vi "Mirror_GUI.vi"(10 "stop 2":refnum<vi>, 11 "GUI_cluster":T1={"Sub Panel"=refnum, "GUIdevice"="Bella_LP_Mode", "CtlRef"=refnum, "user event out"=refnum}) -> ()   [LabVIEW 2011]
uses:
  Controls/GUI_cluster.ctl
  Controls/eventtypdef.ctl
  GUI_Template/GUI_master/tcp new data cluster.ctl
  General-Controler/firstCall_TypDef.ctl
panel:
  out "UDP error message":string
  out "status ref":refnum<vi>[](array[refnum])
  out "pathRef":refnum<vi>[](array[refnum])
  in  "pushSave":bool
  out "Page Label":string="StagingTRA1"
  in  "save::4":bool caption="save"
  in  "save::3":bool caption="save"
  in  "save::2":bool caption="save"
  in  "save::1":bool caption="save"
  in  "LocalSavingPath::4":path=path "Z:/5_resources/StagingResources/TRAposition/testNEW" caption="LocalSavingPath::1"
  in  "LocalSavingPath::3":path=path "Z:/5_resources/StagingResources/TRAposition/testNEW" caption="LocalSavingPath::1"
  in  "LocalSavingPath::2":path=path "Z:/5_resources/StagingResources/TRAposition/testNEW" caption="LocalSavingPath::1"
  in  "LocalSavingPath::1":path=path "Z:/5_resources/StagingResources/TRAposition/testNEW"
  in  "save":bool
  out "GUIdevice 3":string="StagingTRA3"
  out "GUIdevice 4":string="TREX TRA1"
  out "error out":errorcluster
  out "GUIdevice 2":string="StagingTRA2"
  in  "Tab Control":T2(tab)
  in  "StepSize::1":dbl=0.01 caption="StepSize" min=-1.0 max=1.0 format="%#_2p"
  in  "Cluster 20":T3
  in  "Y":T4={"position::1"=2.74161, "Channel::1"=enum."Axis 2", "Status::1"=enum."DISABLE"} {"position::1" min=0.0 max=6.0 format="%#_8g"}
  in  "X":T5={"position::1"=3.02685, "Channel::1"=enum."Axis 1", "Status::1"=enum."DISABLE"} {"position::1" min=0.0 max=6.0 format="%#_8g"}
  in  "Cluster 40":T6
  in  "Cluster 50":T7
  in  "Cluster 30":T8
  out "device status::1":string="Initialized" caption="Device status"
  in  "<command>::1":bool
  in  "StepSize::2":dbl=0.01 caption="StepSize" min=-1.0 max=1.0 format="%#_2p"
  in  "Cluster 23":T9
  in  "Y":T10={"position::2"=3.24237, "Channel::2"=enum."Axis 2", "Status::2"=enum."DISABLE"} {"position::2" min=0.0 max=6.0 format="%#_8g"}
  in  "X":T11={"position::2"=2.27011, "Channel::2"=enum."Axis 1", "Status::2"=enum."DISABLE"} {"position::2" min=0.0 max=6.0 format="%#_8g"}
  in  "Cluster 43":T12
  in  "Cluster 53":T13
  in  "Cluster 33":T14
  out "device status::2":string="Initialized" caption="Device status"
  in  "<command>::2":bool
  in  "StepSize::3":dbl=0.01 caption="StepSize" min=-1.0 max=1.0 format="%#_2p"
  in  "Cluster 22":T15
  in  "Y":T16={"position::3"=5.00224, "Channel::3"=enum."Axis 2", "Status::3"=enum."DISABLE"} {"position::3" min=0.0 max=0.0 format="%#_8g"}
  in  "X":T17={"position::3"=1.52721, "Channel::3"=enum."Axis 1", "Status::3"=enum."DISABLE"} {"position::3" min=0.0 max=0.0 format="%#_8g"}
  in  "Cluster 42":T18
  in  "Cluster 52":T19
  in  "Cluster 32":T20
  out "device status::3":string="Initialized" caption="Device status"
  in  "<command>::3":bool
  in  "StepSize::4":dbl=0.01 caption="StepSize" min=-1.0 max=1.0 format="%#_2p"
  in  "Cluster 21":T21
  in  "Y":T22={"position::4"=4.68088, "Channel::4"=enum."Axis 2", "Status::4"=enum."DISABLE"} {"position::4" min=0.0 max=6.0 format="%#_8g"}
  in  "X":T23={"position::4"=0.99394, "Channel::4"=enum."Axis 1", "Status::4"=enum."DISABLE"} {"position::4" min=0.0 max=6.0 format="%#_8g"}
  in  "Cluster 41":T24
  in  "Cluster 51":T25
  in  "Cluster 31":T26
  out "device status::4":string="Initialized" caption="Device status"
  in  "<command>::4":bool
  in  "Mirror":T27(ring)
  out "GUIdevice 1":string="StagingTRA1"
  in  "stop":bool
  in  "Refresh Button":bool
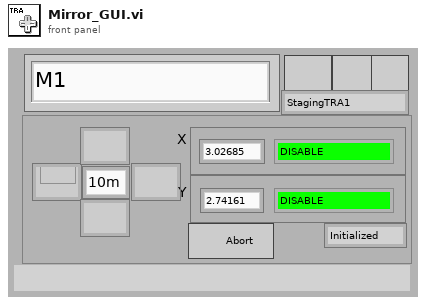
[diagram p1: front panel]
types:
  T1 = typedef "GUI_cluster.ctl" = cluster{"Sub Panel":refnum<vi>, "GUIdevice":string, "CtlRef":refnum<vi>, "user event out":refnum<user-event>}
  T2 = enum32{"StagingTRA1", "StagingTRA2", "StagingTRA3", "TREX TRA1"}
  T3 = cluster{"relativeMovePos::1":bool, "Channel::1":enum16{"Axis 1", "Axis 3", "Axis 5"}}
  T4 = cluster{"position::1":dbl, "Channel::1":enum16{"Axis 2", "Axis 4", "Axis 6"}, "Status::1":enum16{"NOT REFERENCED", "CONFIGURATION", "HOMING", "MOVING", "READY", "DISABLE", "JOGGING"}}
  T5 = cluster{"position::1":dbl, "Channel::1":enum16{"Axis 1", "Axis 3", "Axis 5"}, "Status::1":enum16{"NOT REFERENCED", "CONFIGURATION", "HOMING", "MOVING", "READY", "DISABLE", "JOGGING"}}
  T6 = cluster{"relativeMovePos::1":bool, "Channel::1":enum16{"Axis 2", "Axis 4", "Axis 6"}}
  T7 = cluster{"relativeMoveNeg::1":bool, "Channel::1":enum16{"Axis 2", "Axis 4", "Axis 6"}}
  T8 = cluster{"relativeMoveNeg::1":bool, "Channel::1":enum16{"Axis 1", "Axis 3", "Axis 5"}}
  T9 = cluster{"relativeMovePos::2":bool, "Channel::2":enum16{"Axis 1", "Axis 3", "Axis 5"}}
  T10 = cluster{"position::2":dbl, "Channel::2":enum16{"Axis 2", "Axis 4", "Axis 6"}, "Status::2":enum16{"NOT REFERENCED", "CONFIGURATION", "HOMING", "MOVING", "READY", "DISABLE", "JOGGING"}}
  T11 = cluster{"position::2":dbl, "Channel::2":enum16{"Axis 1", "Axis 3", "Axis 5"}, "Status::2":enum16{"NOT REFERENCED", "CONFIGURATION", "HOMING", "MOVING", "READY", "DISABLE", "JOGGING"}}
  T12 = cluster{"relativeMovePos::2":bool, "Channel::2":enum16{"Axis 2", "Axis 4", "Axis 6"}}
  T13 = cluster{"relativeMoveNeg::2":bool, "Channel::2":enum16{"Axis 2", "Axis 4", "Axis 6"}}
  T14 = cluster{"relativeMoveNeg::2":bool, "Channel::2":enum16{"Axis 1", "Axis 3", "Axis 5"}}
  T15 = cluster{"relativeMovePos::3":bool, "Channel::3":enum16{"Axis 1", "Axis 3", "Axis 5"}}
  T16 = cluster{"position::3":dbl, "Channel::3":enum16{"Axis 2", "Axis 4", "Axis 6"}, "Status::3":enum16{"NOT REFERENCED", "CONFIGURATION", "HOMING", "MOVING", "READY", "DISABLE", "JOGGING"}}
  T17 = cluster{"position::3":dbl, "Channel::3":enum16{"Axis 1", "Axis 3", "Axis 5"}, "Status::3":enum16{"NOT REFERENCED", "CONFIGURATION", "HOMING", "MOVING", "READY", "DISABLE", "JOGGING"}}
  T18 = cluster{"relativeMovePos::3":bool, "Channel::3":enum16{"Axis 2", "Axis 4", "Axis 6"}}
  T19 = cluster{"relativeMoveNeg::3":bool, "Channel::3":enum16{"Axis 2", "Axis 4", "Axis 6"}}
  T20 = cluster{"relativeMoveNeg::3":bool, "Channel::3":enum16{"Axis 1", "Axis 3", "Axis 5"}}
  T21 = cluster{"relativeMovePos::4":bool, "Channel::4":enum16{"Axis 1", "Axis 3", "Axis 5"}}
  T22 = cluster{"position::4":dbl, "Channel::4":enum16{"Axis 2", "Axis 4", "Axis 6"}, "Status::4":enum16{"NOT REFERENCED", "CONFIGURATION", "HOMING", "MOVING", "READY", "DISABLE", "JOGGING"}}
  T23 = cluster{"position::4":dbl, "Channel::4":enum16{"Axis 1", "Axis 3", "Axis 5"}, "Status::4":enum16{"NOT REFERENCED", "CONFIGURATION", "HOMING", "MOVING", "READY", "DISABLE", "JOGGING"}}
  T24 = cluster{"relativeMovePos::4":bool, "Channel::4":enum16{"Axis 2", "Axis 4", "Axis 6"}}
  T25 = cluster{"relativeMoveNeg::4":bool, "Channel::4":enum16{"Axis 2", "Axis 4", "Axis 6"}}
  T26 = cluster{"relativeMoveNeg::4":bool, "Channel::4":enum16{"Axis 1", "Axis 3", "Axis 5"}}
  T27 = enum16{"M1", "BS", "M3", "OAP1", "M4", "OAP2", "M5", "n/a", "n/a ", "M20", "SIM", "M22"}
  T28 = typedef "eventtypdef.ctl" = cluster{"label":string, "Sub Panel":refnum<vi>, "CtlRef":refnum<vi>, "This VI":refnum<vi>}
  T29 = typedef "tcp new data cluster.ctl" = cluster{"EventEnum":enum16{"new data", "connection status update"}, "Device name":string}
  T30 = typedef "firstCall_TypDef.ctl" = enum16{"reset", "read"}
  T31 = typedef "LVFontTypeDef.ctl" = cluster{"Font Name":string, "Size":u16, "Bold":bool, "Italic":bool, "Underline":bool, "Strikeout":bool, "Color":u32}
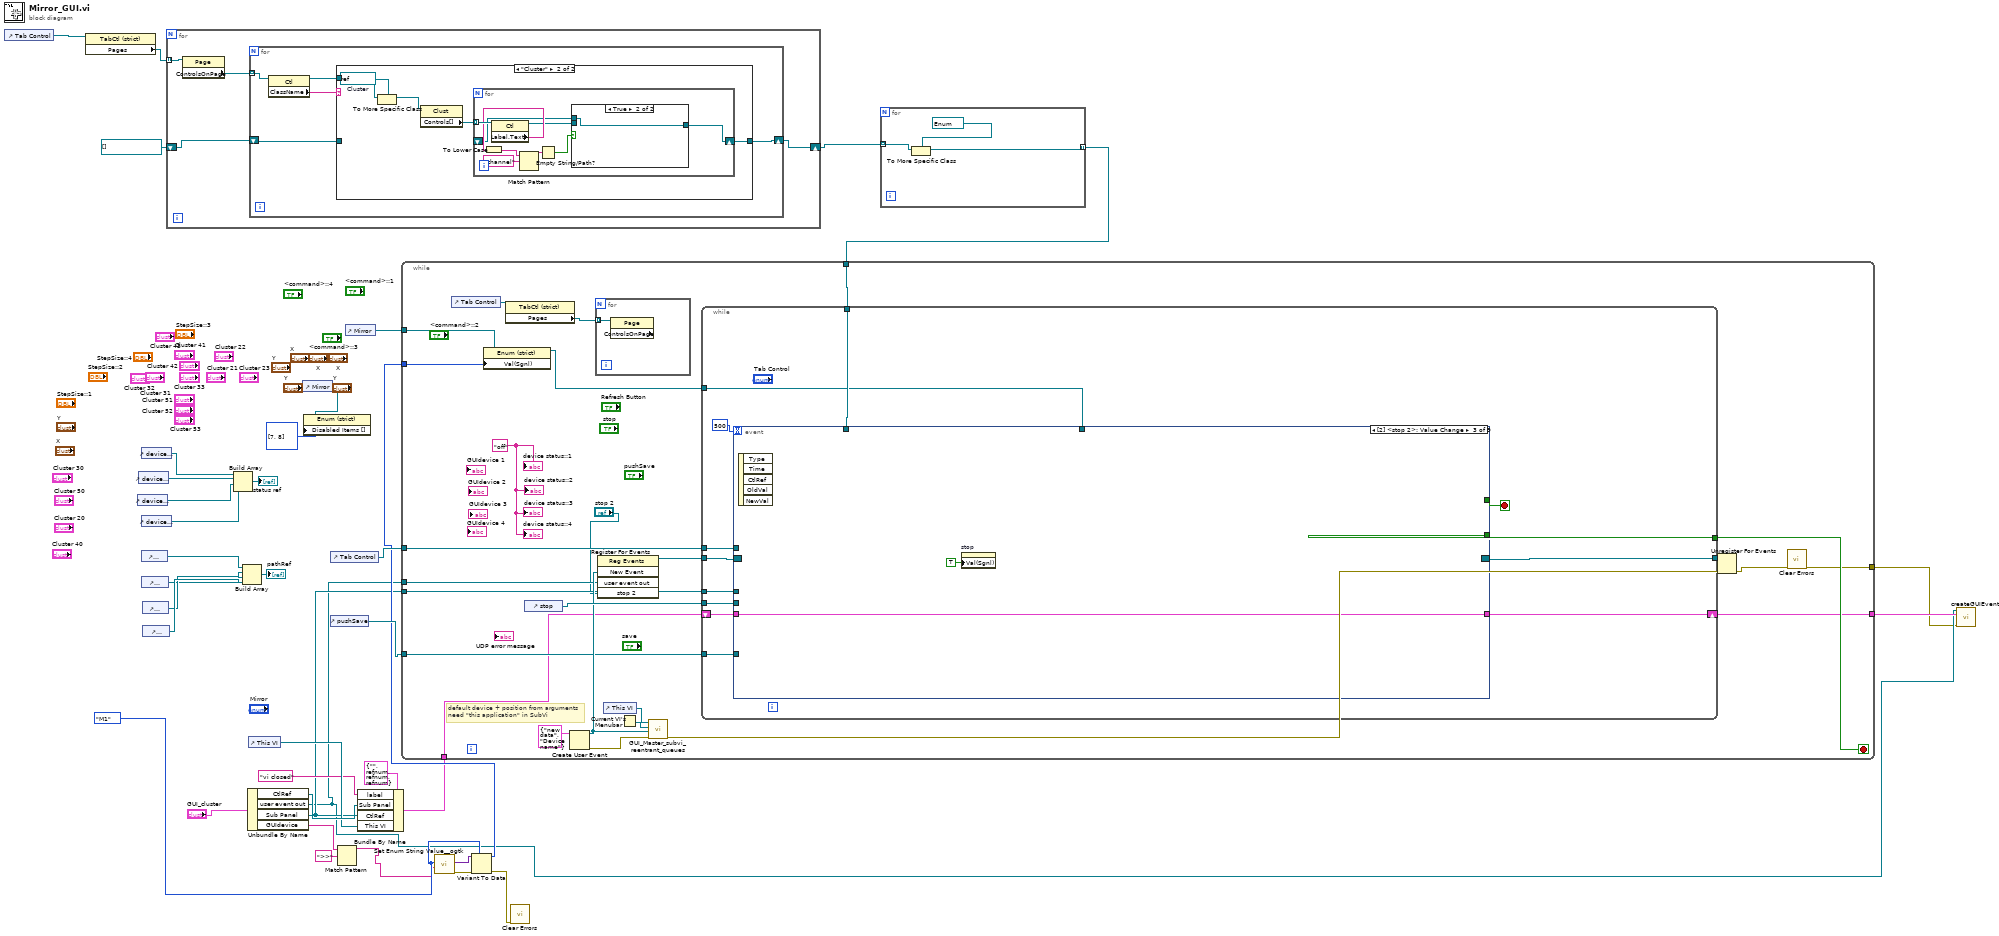
[diagram p0: block diagram]
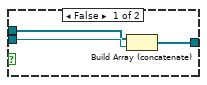
[diagram p3: hidden frame]
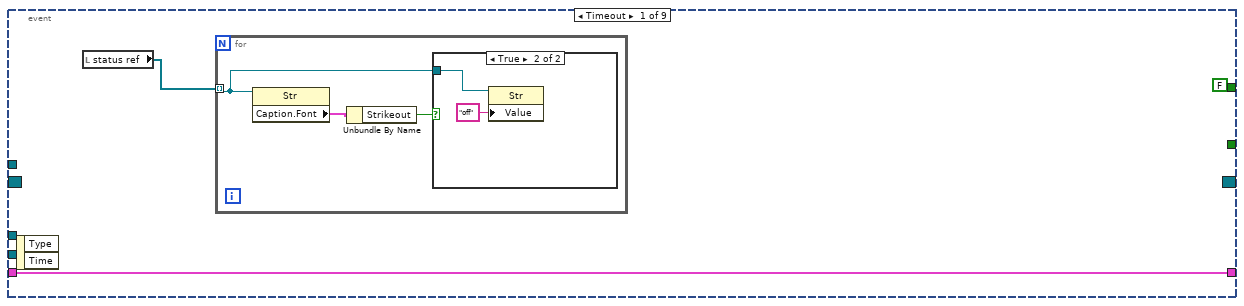
[diagram p4: hidden frame]
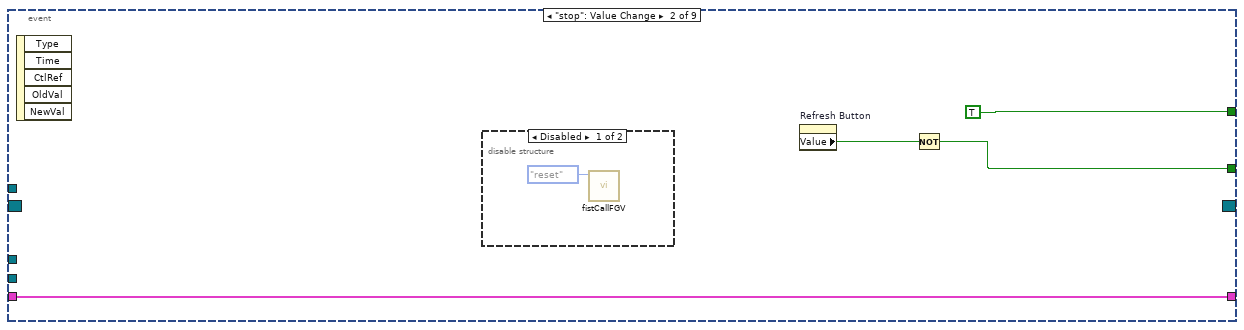
[diagram p6: hidden frame]
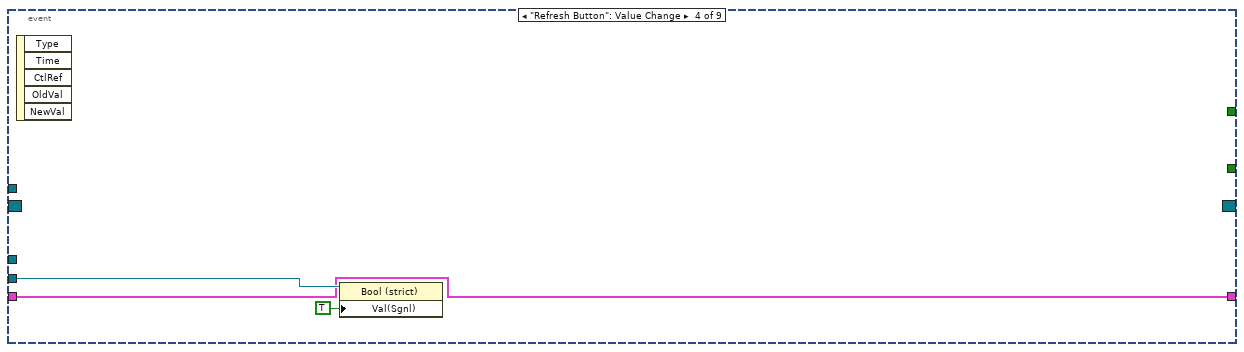
[diagram p8: hidden frame]
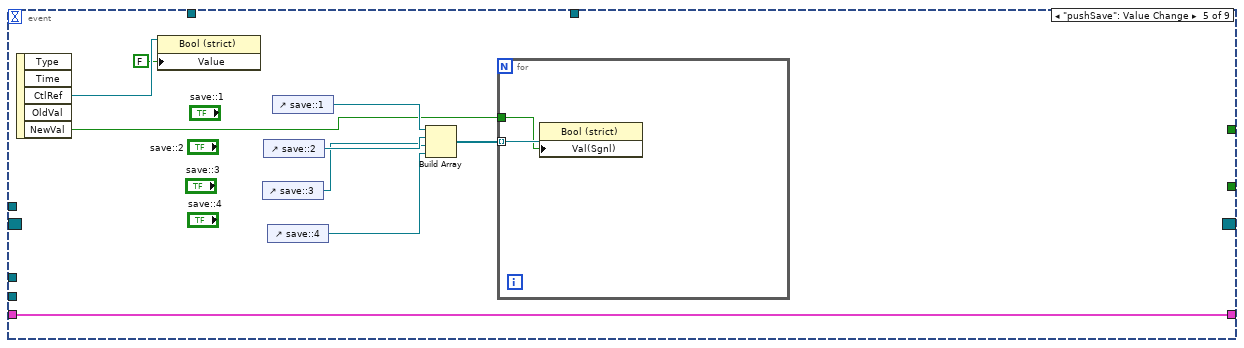
[diagram p9: hidden frame]
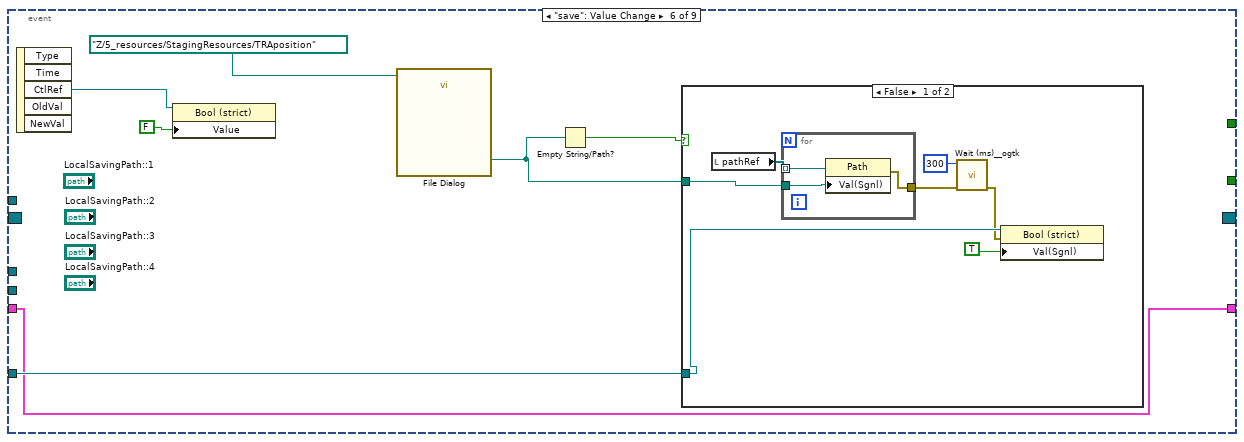
[diagram p10: hidden frame]
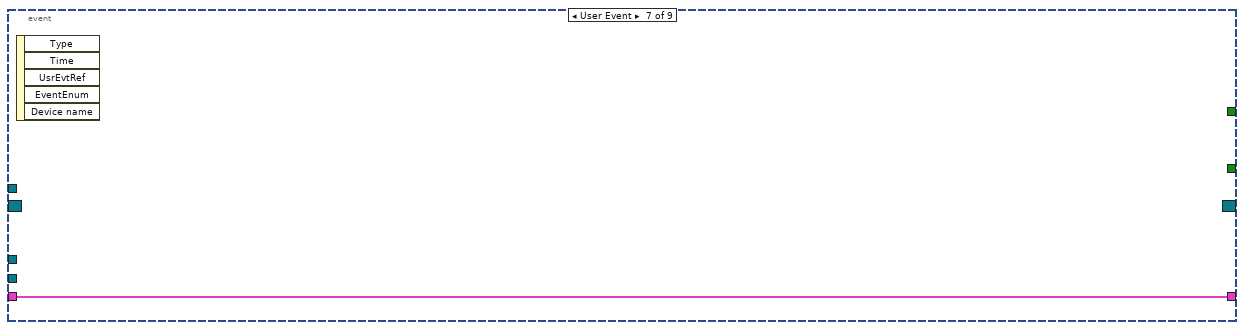
[diagram p12: hidden frame]
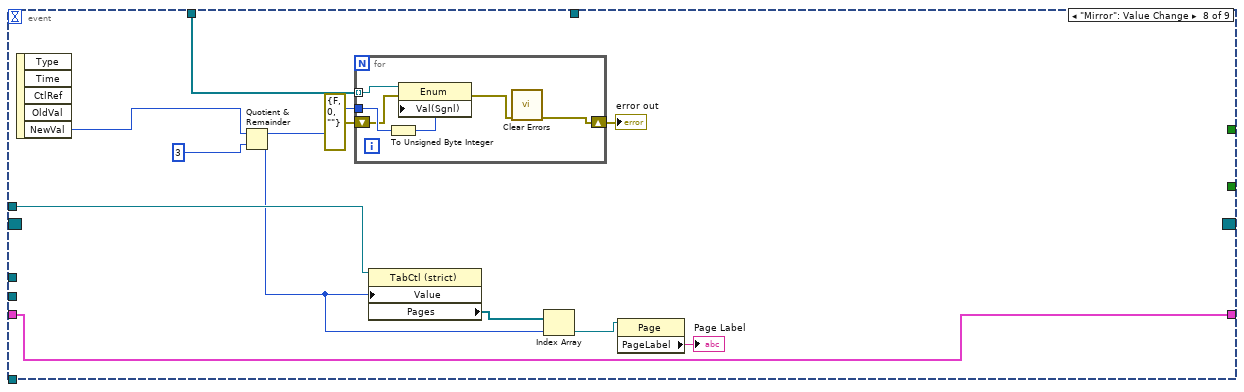
[diagram p13: hidden frame]
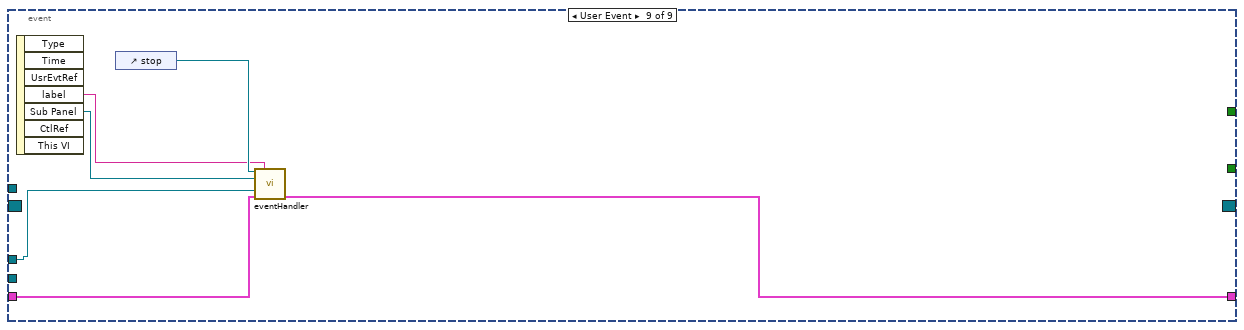
[diagram p14: hidden frame]
diagram:
  w11 = T27."M1" ("Value (Signaling)")
  n1 = control-ref of="Tab Control"() -> (w38:refnum<vi>)
  n2 = property class="TabCtl (strict)"(reference=w38) -> ("Pages"=w37:refnum<vi>[])  [unwired: 1 in, 2 out]
  n3 = control-ref of="device status::3"() -> (w21:refnum<vi>)
  n4 = control-ref of="device status::2"() -> (w22:refnum<vi>)
  n5 = control-ref of="device status::1"() -> (w23:refnum<vi>)
  n6 = control-ref of="LocalSavingPath::1"() -> (w26:refnum<vi>)
  n7 = control-ref of="device status::4"() -> (w20:refnum<vi>)
  n8 = control-ref of="LocalSavingPath::2"() -> (w27:refnum<vi>)
  n9 = control-ref of="LocalSavingPath::3"() -> (w28:refnum<vi>)
  n10 = control-ref of="LocalSavingPath::4"() -> (w29:refnum<vi>)
  n11 = for {
    tunnel: w37 -> [w42] mode=indexing
    shift-right: [w40] -> w35
    shift-left: refnum<vi>[] [] -> [w39]
    n12 = property class="Page"(reference=w42) -> ("ControlsOnPage"=w41:refnum<vi>[])  [unwired: 1 in, 2 out]
    n13 = for {
      tunnel: w41 -> [w47] mode=indexing
      shift-right: [w44] -> w40
      shift-left: w39 -> [w43]
      n14 = property class="Ctl"(reference=w47) -> (reference out=w45:refnum<vi>, "ClassName"=w46:string)  [unwired: 1 in, 1 out]
      n15 = case shown="\"Cluster\"" w46 {
        tunnel: w45 -> [_ w53]
        tunnel: [w48 w49] -> w44
        tunnel: w43 -> [w48 _]
        frame "False", Default {
        }
        frame "Cluster" {
          w52 = refnum<vi> refnum  # Cluster
          n16 = To More Specific Class(target class=w52, reference=w53) -> (specific class reference=w51:refnum<vi>)  [unwired: 1 in, 1 out]
          n17 = property class="Clust"(reference=w51) -> ("Controls[]"=w50:refnum<vi>[])  [unwired: 1 in, 2 out]
          n18 = for {
            tunnel: w50 -> [w62] mode=indexing
            shift-right: [w55] -> w49
            shift-left: _ -> [w54]
            n19 = property class="Ctl"(reference=w62) -> (reference out=w56:refnum<vi>, "Label.Text"=w60:string)  [unwired: 1 in, 1 out]
            n20 = To Lower Case(string=w60) -> (all lower case string=w59:string)
            n21 = Match Pattern(string=w59, regular expression="channel") -> (match substring=w58:string)  [unwired: 1 in, 3 out]
            n22 = Empty String/Path?(string/path=w58) -> (empty?=w57:bool)
            n23 = case shown="True" w57 {
              tunnel: w56 -> [w65 _]
              tunnel: [w64 w66] -> w55
              tunnel: w54 -> [w63 w66]
              frame False {
                n24 = Build Array (concatenate)(w63, w65) -> (w64:refnum<vi>[])
              }
              frame True {
              }
            }
          }
        }
      }
    }
  }
  n25 = Build Array(w23, w22, w21, w20) -> (→"status ref":refnum<vi>[])
  n26 = Build Array(w26, w27, w28, w29) -> (→"pathRef":refnum<vi>[])
  n27 = Unbundle By Name("GUI_cluster") -> ("CtlRef"=w17:refnum<vi>, "user event out"=w2:refnum<user-event>, "Sub Panel"=w5:refnum<vi>, "GUIdevice"=w14:string)
  n28 = control-ref of="This VI"() -> (w16:refnum<vi>)
  n29 = control-ref of="Mirror"() -> (w31:refnum<vi>)
  n30 = property class="Enum (strict)"(reference=w31, "Disabled Items []"=i32[] [7, 8]) -> ()  [unwired: 1 in, 2 out]
  n31 = control-ref of="Tab Control"() -> (w33:refnum<vi>)
  n32 = control-ref of="pushSave"() -> (w24:refnum<vi>)
  n33 = Match Pattern(string=w14, regular expression=">>") -> (before substring=w7:string)  [unwired: 1 in, 3 out]
  n34 = control-ref of="Mirror"() -> (w30:refnum<vi>)
  n35 = Bundle By Name(cluster=T28 {"label"="", "Sub Panel"=refnum, "CtlRef"=refnum, "This VI"=refnum} ("event data"), "label"="vi closed", "Sub Panel"=w5, "CtlRef"=w17, "This VI"=w16) -> (w3:T28)
  n36 = call <userlib>:"Set Enum String Value__ogtk.vi"("String Value"=w7, "Default Enum Value"=w11) -> ("error out"=w8:errorcluster, "Enum"=w12:variant)  [unwired: 8 in]
  n37 = Variant To Data(error in=w8, type=w11, Variant=w12) -> (data=w10:T27, error out=w9:errorcluster)
  n38 = call <vilib>:"Clear Errors.vi"("error in (no error)"=w9) -> ()  [unwired: 6 in, 1 out]
  n39 = for {
    tunnel: w35 -> [w69] mode=indexing
    tunnel: [w68] -> w34 mode=indexing
    n40 = To More Specific Class(target class=refnum<vi> refnum ("Channel::2"), reference=w69) -> (specific class reference=w68:refnum<vi>)  [unwired: 1 in, 1 out]
  }
  n41 = while {
    tunnel: w34 -> [w82]
    tunnel: w33 -> [w81]
    tunnel: w30 -> [w80]
    tunnel: w24 -> [w79]
    tunnel: [w77] -> w1
    tunnel: w2 -> [w76]
    tunnel: w10 -> [w75]
    tunnel: w5 -> [w74]
    tunnel: w3 -> [w72]
    tunnel: [w71] -> w4
    stop <- w93 stop-if-true
    w78 = "off" ("device status::1")
    # "default device + position from arguments\nneed \"this application\" in SubVi"
    n42 = control-ref of="Tab Control"() -> (w84:refnum<vi>)
    n43 = property class="Enum (strict)"(reference=w80, "Val(Sgnl)"=w75) -> (reference out=w73:refnum<vi>)  [unwired: 1 in, 1 out]
    n44 = property class="TabCtl (strict)"(reference=w84) -> ("Pages"=w83:refnum<vi>[])  [unwired: 1 in, 2 out]
    n45 = control-ref of="stop"() -> (w92:refnum<vi>)
    n46 = Create User Event(user event datatype=T29 {"EventEnum"=enum."new data", "Device name"="Device name"} ("New Event")) -> (user event=w87:refnum<user-event>, error out=w88:errorcluster)  [unwired: 1 in]
    n47 = for {
      tunnel: w83 -> [w96] mode=indexing
      n48 = property class="Page" props=["ControlsOnPage"](reference=w96) -> ()  [unwired: 1 in, 3 out]
    }
    n49 = register-events(w87, w76, "stop 2") -> (reference out=w95:refnum<event-registration>)  [unwired: 2 in, 1 out]
    n50 = control-ref of="This VI"() -> (w91:refnum<vi>)
    n51 = Current VI's Menubar() -> (w90:refnum<k9>)
    n52 = call "GUI_Master_subvi_reentrant_queues.vi"("error in (no error)"=w88, "tcp data event"=w87, "Caller menu reference"=w90, "Caller VI ref"=w91) -> ("error out"=w86:errorcluster)  [unwired: 7 in]
    n53 = while {
      tunnel: w95 -> [w109]
      tunnel: [w108] -> w94
      tunnel: [w106] -> w93
      tunnel: w92 -> [w105]
      tunnel: w82 -> [w104]
      tunnel: w81 -> [w103]
      tunnel: w79 -> [w102]
      tunnel: w74 -> [w100]
      tunnel: w73 -> [w99]
      shift-right: [w97] -> w71
      shift-left: w72 -> [w98]
      stop <- w107 stop-if-true
      n54 = event shown="[2] <stop 2>: Value Change" {
        selector: w109 -> [_ _ _ _ _ _ _ _ _]
        dyn-events: [_ _ _ _ _ _ _ _ _] -> w108
        timeout: 500 -> [_ _ _ _ _ _ _ _ _]
        tunnel: [FALSE TRUE _ _ _ _ _ _ _] -> w107
        tunnel: [_ w119 _ _ _ _ _ _ _] -> w106
        tunnel: w105 -> [_ _ _ w127 _ _ _ _ _]
        tunnel: w104 -> [_ _ _ _ _ _ _ w168 _]
        tunnel: w103 -> [_ _ _ _ _ _ _ w162 _]
        tunnel: w102 -> [_ _ _ _ _ w142 _ _ _]
        tunnel: w100 -> [_ _ _ _ _ _ _ _ w177]
        tunnel: w99 -> [_ _ _ _ _ _ _ _ _]
        tunnel: w98 -> [w110 w118 w124 w125 w128 w139 w156 w157 w176]
        tunnel: [w110 w118 w124 w125 w128 w139 w156 w157 w175] -> w97
        event Timeout {
          n55 = event-data() -> ()  [unwired: 1 in, 2 out]
          n56 = local read "status ref"() -> (w111:refnum<vi>[])
          n57 = for {
            tunnel: w111 -> [w113] mode=indexing
            n58 = property class="Str"(reference=w113) -> ("Caption.Font"=w115:T31)  [unwired: 1 in, 2 out]
            n59 = Unbundle By Name(w115) -> ("Strikeout"=w114:bool)
            n60 = case shown="True" w114 {
              tunnel: w113 -> [_ w117]
              frame False {
              }
              frame True {
                n61 = property class="Str"(reference=w117, "Value"="off") -> ()  [unwired: 1 in, 2 out]
              }
            }
          }
        }
        event "stop": Value Change {
          n62 = event-data() -> ()  [unwired: 1 in, 5 out]
          n63 = disable-structure shown="Disabled" {
            frame Disabled {
              n64 = call "fistCallFGV.vi"("Function"=firstCall_TypDef."reset") -> ()  [unwired: 9 in, 2 out]
            }
            frame Enabled {
            }
          }
          n65 = property on="Refresh Button" class="Bool (strict)"() -> ("Value"=w120:bool)  [unwired: 2 in, 2 out]
          n66 = Not(x=w120) -> (.not. x?=w119:bool)
        }
        event Value Change {
          n67 = event-data() -> ()  [unwired: 1 in, 5 out]
          n68 = property on="stop" class="Bool (strict)"("Val(Sgnl)"=TRUE ("Value (Signaling)")) -> ()  [unwired: 2 in, 2 out]
        }
        event "Refresh Button": Value Change {
          n69 = event-data() -> ()  [unwired: 1 in, 5 out]
          n70 = property class="Bool (strict)"(reference=w127, "Val(Sgnl)"=TRUE ("Value (Signaling)")) -> ()  [unwired: 1 in, 2 out]
        }
        event "pushSave": Value Change {
          n71 = event-data() -> ("CtlRef"=w130:refnum<vi>, "NewVal"=w131:bool)  [unwired: 1 in, 3 out]
          n72 = property class="Bool (strict)"(reference=w130, "Value"=FALSE) -> ()  [unwired: 1 in, 2 out]
          n73 = control-ref of="save::3"() -> (w134:refnum<vi>)
          n74 = control-ref of="save::2"() -> (w135:refnum<vi>)
          n75 = control-ref of="save::4"() -> (w133:refnum<vi>)
          n76 = control-ref of="save::1"() -> (w136:refnum<vi>)
          n77 = Build Array(w136, w135, w134, w133) -> (w132:refnum<vi>[])
          n78 = for {
            tunnel: w132 -> [w138] mode=indexing
            tunnel: w131 -> [w137]
            n79 = property class="Bool (strict)"(reference=w138, "Val(Sgnl)"=w137) -> ()  [unwired: 1 in, 2 out]
          }
        }
        event "save": Value Change {
          n80 = event-data() -> ("CtlRef"=w141:refnum<vi>)  [unwired: 1 in, 4 out]
          n81 = property class="Bool (strict)"(reference=w141, "Value"=FALSE) -> ()  [unwired: 1 in, 2 out]
          n82 = call "File Dialog"("start path"=path "Z:/5_resources/StagingResources/TRAposition") -> ("selected path"=w144:path)  [unwired: 11 in, 3 out]
          n83 = Empty String/Path?(string/path=w144) -> (empty?=w143:bool)
          n84 = case shown="False" w143 {
            tunnel: w144 -> [w152 _]
            tunnel: w142 -> [w148 _]
            frame False {
              n85 = local read "pathRef"() -> (w151:refnum<vi>[])
              n86 = for {
                tunnel: w151 -> [w155] mode=indexing
                tunnel: w152 -> [w154]
                tunnel: [w153] -> w150
                n87 = property class="Path"(reference=w155, "Val(Sgnl)"=w154) -> (error out=w153:errorcluster)  [unwired: 1 in, 1 out]
              }
              n88 = call <userlib>:"Wait (ms)__ogtk.vi"("error in (no error)"=w150, "milliseconds to wait"=u32 300) -> ("error out"=w147:errorcluster)  [unwired: 8 in, 1 out]
              n89 = property class="Bool (strict)"(reference=w148, error in=w147, "Val(Sgnl)"=TRUE) -> ()  [unwired: 2 out]
            }
            frame True {
            }
          }
        }
        event User Event {
          n90 = event-data() -> ()  [unwired: 1 in, 5 out]
        }
        event "Mirror": Value Change {
          n91 = event-data() -> ("NewVal"=w167:T27)  [unwired: 1 in, 4 out]
          n92 = Quotient & Remainder(x=w167, y=3) -> (x-y*floor(x/y)=w165:i32, floor(x/y)=w160:i32)
          n93 = for {
            tunnel: w168 -> [w174] mode=indexing
            tunnel: w165 -> [w172]
            shift-right: [w170] -> w163
            shift-left: errorcluster {"status"=FALSE, "code"=0, "source"=""} ("error out") -> [w169]
            n94 = To Unsigned Byte Integer(number=w172) -> (unsigned 8bit integer=w171:u8)
            n95 = property class="Enum"(reference=w174, error in=w169, "Val(Sgnl)"=w171) -> (error out=w173:errorcluster)  [unwired: 1 out]
            n96 = call <vilib>:"Clear Errors.vi"("error in (no error)"=w173) -> ("error out"=w170:errorcluster)  [unwired: 6 in]
          }
          "error out" <- w163
          n97 = property class="TabCtl (strict)"(reference=w162, "Value"=w160) -> ("Pages"=w161:refnum<vi>[])  [unwired: 1 in, 2 out]
          n98 = Index Array(array=w161, index=w160) -> (element=w159:refnum<vi>)
          n99 = property class="Page"(reference=w159) -> ("PageLabel"=→"Page Label":string)  [unwired: 1 in, 2 out]
        }
        event User Event {
          n100 = event-data() -> ("label"=w179:string, "Sub Panel"=w178:refnum<vi>)  [unwired: 1 in, 5 out]
          n101 = control-ref of="stop"() -> (w180:refnum<vi>)
          n102 = call "eventHandler.vi"("Boolean in"=w180, "label"=w179, "Sub Panel 2"=w178, "Sub Panel"=w177, "event data in"=w176) -> ("event data out"=w175:T28)  [unwired: 10 in]
        }
      }
    }
    n103 = Unregister For Events(event registration refnum=w94, error in=w86) -> (error out=w85:errorcluster)
    n104 = call <vilib>:"Clear Errors.vi"("error in (no error)"=w85) -> ("error out"=w77:errorcluster)  [unwired: 6 in]
    "device status::1" <- w78
    "device status::2" <- w78
    "device status::3" <- w78
    "device status::4" <- w78
  }
  n105 = call "createGUIEvent.vi"("error in (no error)"=w1, "event data"=w4, "User Event in"=w2) -> ()  [unwired: 9 in]
